vi "总磷氨氮插入数据.vi"(0 "table":string, 5 "data":T2={"时间标识"=timestamp(0 s since 1904-01-01), "测量模式"=enum."水样测试", "数据标记表"="N", "监测值"=0.0, "单位"=0, "数据标识"="", "因子编码"=0, "标样参考值"=0.0, "F0"=0.0, "F1"=0.0, "F2"=0.0, "F3"=0.0, "F4"=0.0, "F5"=0.0, "F6"=0.0, "F7"=0.0, "X"=0.0, "温度"=0.0, "湿度"=0.0, "量程标识"="", "SN"="", "跨度值"=0.0, "X1"=0.0} {"单位" items=["μg/L", "mg/L", "ppm", "mg/m3", "cm", "ppb", "μg/m3", "%", "nmol/mol", "μmol/mol", "MPN/L", "MPN/100ml", "ng/m3", "NTU", "无量纲", "ms/cm", "μs/cm"]}, 7 "关键参数":T1, 11 "error in (no error)":errorcluster) -> (15 "error out":errorcluster)   [LabVIEW 2016, in "斯坦道总磷总氮.lvlib"]
uses:
  <vilib>/Utility/error.llb/DialogType.ctl
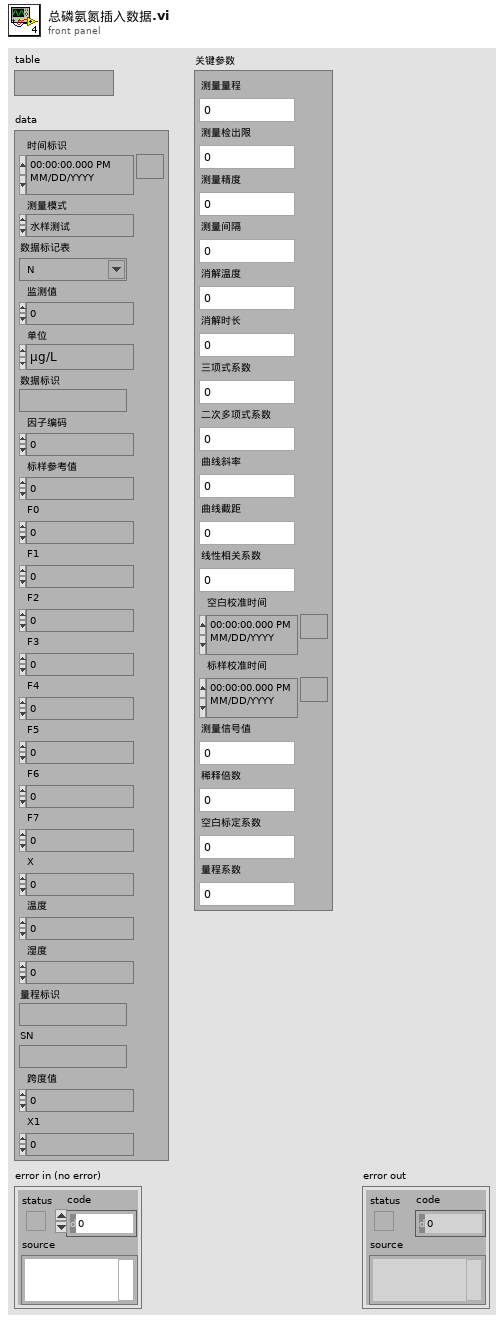
[diagram p1: front panel]
types:
  T1 = typedef "斯坦道总磷总氮.lvlib/关键参数.ctl" = cluster{"测量量程":sgl, "测量检出限":sgl, "测量精度":sgl, "测量间隔":sgl, "消解温度":sgl, "消解时长":sgl, "三项式系数":sgl, "二次多项式系数":sgl, "曲线斜率":sgl, "曲线截距":sgl, "线性相关系数":sgl, "空白校准时间":timestamp, "标样校准时间":timestamp, "测量信号值":sgl, "稀释倍数":sgl, "空白标定系数":sgl, "量程系数":sgl}
  T2 = cluster{"时间标识":timestamp, "测量模式":enum16{"维护数据", "水样测试", "标样核查", "零点核查", "跨度核查", "空白测试", "平行样测试", "加标回收", "空白校准", "标样校准", "初始化（清洗）", "快捷测试"}, "数据标记表":string, "监测值":sgl, "单位":u16, "数据标识":string, "因子编码":u32, "标样参考值":sgl, "F0":sgl, "F1":sgl, "F2":sgl, "F3":sgl, "F4":sgl, "F5":sgl, "F6":sgl, "F7":sgl, "X":sgl, "温度":sgl, "湿度":sgl, "量程标识":string, "SN":string, "跨度值":sgl, "X1":sgl}
  T3 = typedef "DialogType.ctl" = u16
  T4 = typedef "营养盐字段定义.ctl" = cluster{"时间":timestamp, "测量模式":string, "数据类型":string, "检测值":sgl, "单位":string, "数据标识":string, "X":sgl, "量程标识":string, "SN":string, "标样参考值":sgl, "跨度值":sgl, "F0":sgl, "F1":sgl, "F2":sgl, "F3":sgl, "F4":sgl, "F5":sgl, "F6":sgl, "F7":sgl, "X1":sgl, "因子编码":string, "温度":sgl, "湿度":sgl, "测量量程":sgl, "测量检出限":sgl, "测量精度":sgl, "测量间隔":sgl, "消解温度":sgl, "消解时长":sgl, "三项式系数":sgl, "二次多项式系数":sgl, "曲线斜率":sgl, "曲线截距":sgl, "线性相关系数":sgl, "空白校准时间":timestamp, "标样校准时间":timestamp, "测量信号值":sgl, "稀释倍数":sgl, "空白标定系数":sgl, "量程系数":sgl, "LastTime":timestamp}
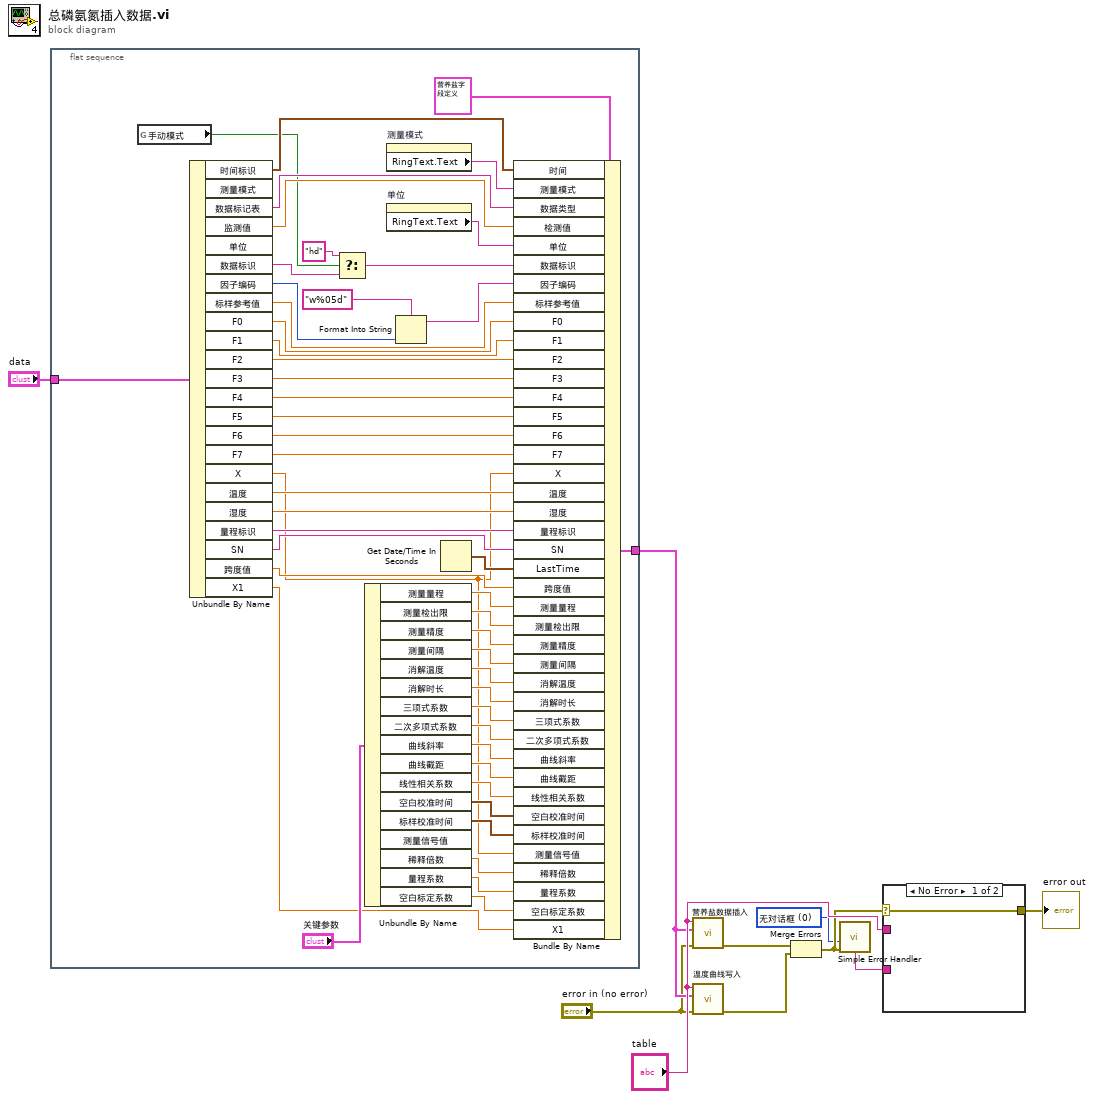
[diagram p0: block diagram]
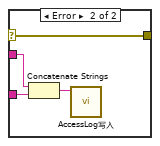
[diagram p2: hidden frame]
diagram:
  w2 = T3 0 items=["无对话框", "确定信息", "继续或停止信息", "确定信息＋警告", "继续/停止+警告"] ("type of dialog (OK msg:1)")
  n1 = flat-sequence {
    tunnel: "data" -> [w40]
    tunnel: [w15] -> w6
    frame #0 {
      n2 = global read "VAR总磷总氮全局变量.vi" "手动模式"() -> (w14:bool)
      n3 = Unbundle By Name(w40) -> ("时间标识"=w59:timestamp, "数据标记表"=w57:string, "监测值"=w56:sgl, "数据标识"=w12:string, "因子编码"=w39:u32, "标样参考值"=w54:sgl, "F0"=w53:sgl, "F1"=w52:sgl, "F2"=w51:sgl, "F3"=w50:sgl, "F4"=w49:sgl, "F5"=w48:sgl, "F6"=w47:sgl, "F7"=w46:sgl, "X"=w19:sgl, "温度"=w45:sgl, "湿度"=w44:sgl, "量程标识"=w43:string, "SN"=w42:string, "跨度值"=w36:sgl, "X1"=w17:sgl)  [unwired: 2 out]
      n4 = Select(t="hd", s=w14, f=w12) -> (s? t:f=w11:string)
      n5 = Unbundle By Name("关键参数") -> ("测量量程"=w34:sgl, "测量检出限"=w33:sgl, "测量精度"=w32:sgl, "测量间隔"=w31:sgl, "消解温度"=w30:sgl, "消解时长"=w29:sgl, "三项式系数"=w28:sgl, "二次多项式系数"=w27:sgl, "曲线斜率"=w26:sgl, "曲线截距"=w25:sgl, "线性相关系数"=w24:sgl, "空白校准时间"=w23:timestamp, "标样校准时间"=w22:timestamp, "稀释倍数"=w21:sgl, "量程系数"=w20:sgl, "空白标定系数"=w18:sgl)  [unwired: 1 out]
      n6 = property on="测量模式" class="Enum (strict)"() -> ("RingText.Text"=w58:string)  [unwired: 2 in, 2 out]
      n7 = property on="单位" class="Ring (strict)"() -> ("RingText.Text"=w55:string)  [unwired: 2 in, 2 out]
      n8 = Format Into String(format string="w%05d" ("格式字符串"), w39) -> (resulting string=w37:string)  [unwired: 2 in, 1 out]
      n9 = Get Date/Time In Seconds() -> (seconds since 1Jan1904=w41:timestamp)
      n10 = Bundle By Name(cluster=T4 {"时间"=timestamp(0 s since 1904-01-01), "测量模式"="水样测试", "数据类型"="N", "检测值"=0.0, "单位"="mg/L", "数据标识"="N", "X"=0.0, "量程标识"="", "SN"="", "标样参考值"=0.0, "跨度值"=0.0, "F0"=0.0, "F1"=0.0, "F2"=0.0, "F3"=0.0, "F4"=0.0, "F5"=0.0, "F6"=0.0, "F7"=0.0, "X1"=0.0, "因子编码"="", "温度"=0.0, "湿度"=0.0, "测量量程"=0.0, "测量检出限"=0.0, "测量精度"=0.0, "测量间隔"=0.0, "消解温度"=0.0, "消解时长"=0.0, "三项式系数"=0.0, "二次多项式系数"=0.0, "曲线斜率"=0.0, "曲线截距"=0.0, "线性相关系数"=0.0, "空白校准时间"=timestamp(0 s since 1904-01-01), "标样校准时间"=timestamp(0 s since 1904-01-01), "测量信号值"=0.0, "稀释倍数"=0.0, "空白标定系数"=0.0, "量程系数"=0.0, "LastTime"=timestamp(0 s since 1904-01-01)} ("data"), "时间"=w59, "测量模式"=w58, "数据类型"=w57, "检测值"=w56, "单位"=w55, "数据标识"=w11, "因子编码"=w37, "标样参考值"=w54, "F0"=w53, "F1"=w52, "F2"=w51, "F3"=w50, "F4"=w49, "F5"=w48, "F6"=w47, "F7"=w46, "X"=w19, "温度"=w45, "湿度"=w44, "量程标识"=w43, "SN"=w42, "LastTime"=w41, "跨度值"=w36, "测量量程"=w34, "测量检出限"=w33, "测量精度"=w32, "测量间隔"=w31, "消解温度"=w30, "消解时长"=w29, "三项式系数"=w28, "二次多项式系数"=w27, "曲线斜率"=w26, "曲线截距"=w25, "线性相关系数"=w24, "空白校准时间"=w23, "标样校准时间"=w22, "测量信号值"=w19, "稀释倍数"=w21, "量程系数"=w20, "空白标定系数"=w18, "X1"=w17) -> (w15:T4)
    }
  }
  n11 = call "营养盐数据插入.vi"("Tabe Name"="table", "data"=w6, "错误输入（无错误）"="error in (no error)") -> ("错误输出"=w8:errorcluster)  [unwired: 7 in]
  n12 = call "温度曲线写入.vi"("error in (no error)"="error in (no error)", "columns"=w6, "table"="table") -> ("错误输出"=w4:errorcluster)  [unwired: 8 in]
  n13 = Merge Errors(w8, w4) -> (w3:errorcluster)
  n14 = call <vilib>:"Simple Error Handler.vi"("type of dialog (OK msg:1)"=w2, "error in (no error)"=w3) -> ("message"=w1:string)  [unwired: 3 in, 4 out]
  n15 = case shown="No Error" w3 {
    selector: w3 -> [w60 w64]
    tunnel: [w60 w64] -> w10
    tunnel: "table" -> [_ w63]
    tunnel: w1 -> [_ w62]
    frame No Error {
    }
    frame Error {
      n16 = Concatenate Strings(w63, w62) -> (w61:string)
      n17 = call "AccessLog写入.vi"("Log"=w61) -> ()  [unwired: 11 in]
    }
  }
  "error out" <- w10
